vi "Set_Pulse.vi"(2 "error in":errorcluster, 3 "Data in":T1) -> (0 "error out":errorcluster, 1 "Data out":T1)   [LabVIEW 2017, in "Steps.lvlib"]
uses:
  Steps.lvlib
  Type_Defs/Data.ctl
  Type_Defs/Diagnostics.ctl
  Type_Defs/Systems.ctl
panel:
  in  "Helical Voltage":dbl[](array[numeric])
  in  "Toroidal Voltage":dbl[](array[numeric])
  in  "Time":dbl[](array[numeric])
  in  "Step Back":bool
  in  "Continue":bool
  # "Set the pulse for the next shot."
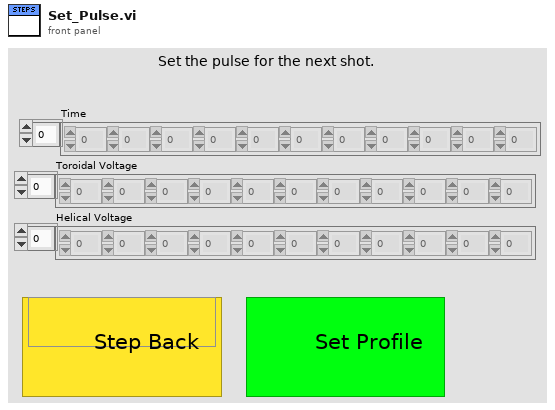
[diagram p1: front panel]
types:
  T1 = typedef "Data.ctl" = cluster{"User Name":string, "Experiment Number":i32, "Start Time":timestamp, "Data":dbl[], "Step Number":i32, "Step Instructions":string, "Diagnostics":T2, "Experiment Purpose":string, "Experiment State":enum16{"Off", "Setting Up", "Ready", "In Progress", "Shutting Down"}, "Systems":T3, "Vacuum Pressure":dbl, "Fieldpoints":cluster{"System Boolean Fieldpoints":cluster{"Compressed Air":refnum<k21>, "T-20kV Power Switch":refnum<k21>, "T-Rectifier":refnum<k21>, "Engage Interlock":refnum<k21>, "Ventilator":refnum<k21>, "Magnetron":refnum<k21>, "H-20kV Power Switch":refnum<k21>, "H-Rectifier":refnum<k21>, "Main Water Pump":refnum<k21>, "WEGA Water Pump":refnum<k21>, "Gas Inlet Valves":refnum<k21>}, "Step Fieldpoints":cluster{"Exhaust Ventillator":refnum<k21>, "Compressed Air":refnum<k21>, "Water Pressure":refnum<k21>, "Interlock":refnum<k21>, "Toroidal Power Supply 1":refnum<k21>, "Toroidal Power Supply 2":refnum<k21>, "Toroidal Rectifier":refnum<k21>, "Helical Power Supply":refnum<k21>, "Helical Rectifier":refnum<k21>, "6kW Magnetron Standby":refnum<k21>, "20kW Magnetron Standby":refnum<k21>}}, "Pressure History":cluster{"Seconds into Experiment":i32[], "Pressure Data":dbl[]}, "Time Computer Control":dbl[], "Toroidal Voltage Computer Control":dbl[], "Helical Voltage Computer Control":dbl[], "Toroidal Current":dbl[], "Toroidal Voltage":dbl[], "Toroidal Current Set Point":dbl[], "Helical Current Set Point":dbl[], "Helical Voltage":dbl[], "Helical Current":dbl[], "Experiment Folder":path, "Run Another Shot?":bool}
  T2 = typedef "Diagnostics.ctl" = cluster{"Langmuir Probe":bool, "Rogowski 1":bool, "Rogowski 2":bool, "Rogowski 3":bool, "B-dot 1":bool, "B-dot 2":bool}
  T3 = typedef "Systems.ctl" = cluster{"Compressed Air":bool, "T-20kV Power Switch":bool, "T-Rectifier":bool, "Engage Interlock":bool, "Ventilator":bool, "Magnetron":bool, "H-20kV Power Switch":bool, "H-Rectifier":bool, "Main Water Pump":bool, "WEGA Water Pump":bool, "Gas Inlet Valves":bool}
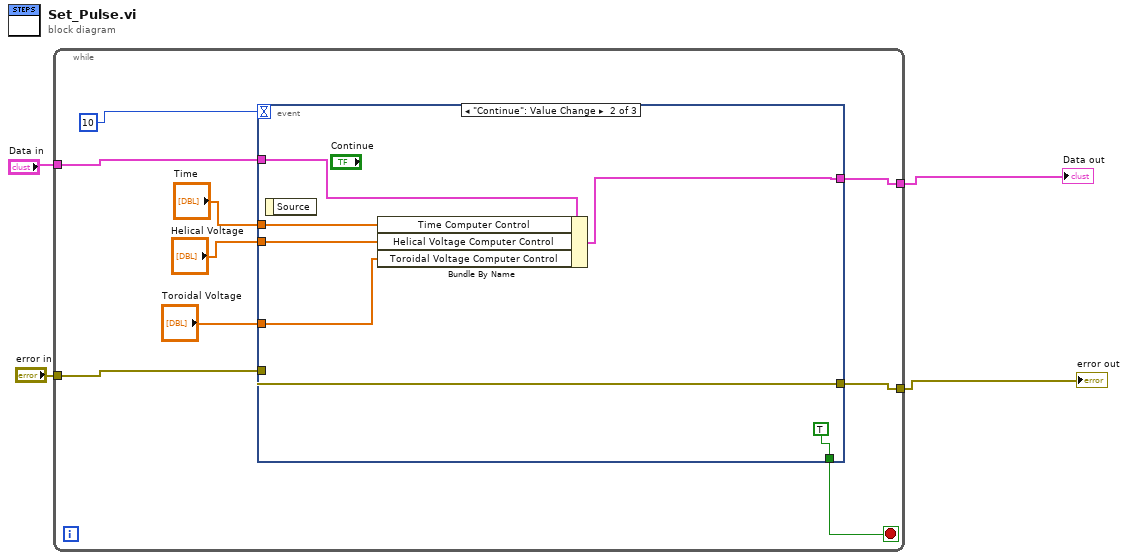
[diagram p0: block diagram]
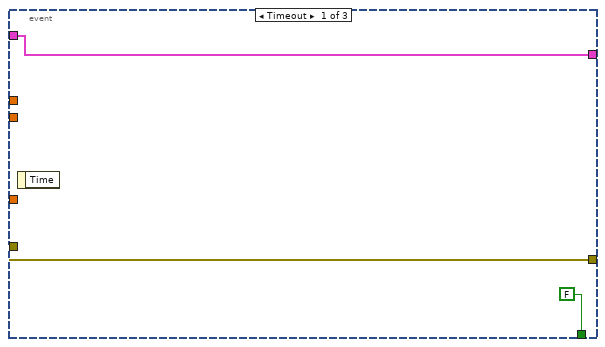
[diagram p2: hidden frame]
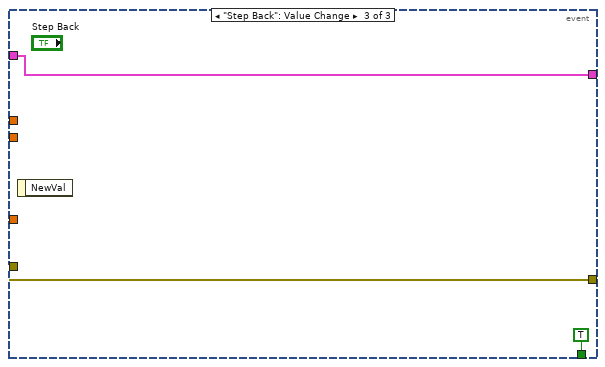
[diagram p3: hidden frame]
diagram:
  n1 = while {
    tunnel: "error in" -> [w13]
    tunnel: [w12] -> w1
    tunnel: [w10] -> w2
    tunnel: "Data in" -> [w9]
    stop <- w11 stop-if-true
    n2 = event shown="[1] \"Continue\": Value Change" {
      selector: _ -> [_ _ _]
      dyn-events: _ -> [_ _ _]
      timeout: 10 -> [_ _ _]
      tunnel: w13 -> [w15 w23 w26]
      tunnel: [w15 w23 w26] -> w12
      tunnel: [FALSE TRUE TRUE] -> w11
      tunnel: [w14 w21 w24] -> w10
      tunnel: w9 -> [w14 w20 w24]
      tunnel: "Time" -> [_ w19 _]
      tunnel: "Helical Voltage" -> [_ w18 _]
      tunnel: "Toroidal Voltage" -> [_ w17 _]
      event Timeout {
        n3 = event-data() -> ()  [unwired: 1 in, 1 out]
      }
      event "Continue": Value Change {
        n4 = event-data() -> ()  [unwired: 1 in, 1 out]
        n5 = Bundle By Name(cluster=w20, "Time Computer Control"=w19, "Helical Voltage Computer Control"=w18, "Toroidal Voltage Computer Control"=w17) -> (w21:T1)
      }
      event "Step Back": Value Change {
        n6 = event-data() -> ()  [unwired: 1 in, 1 out]
      }
    }
  }
  "error out" <- w1
  "Data out" <- w2
